vi "Modifying the Color Table2可加入多个颜色.vi"(7 "停止":bool, 8 "更新刻度颜色":bool, 9 "Z标尺.刻度值[]":cluster{"数值输入控件":dbl, "颜色盒":u32}[](array[cluster])=[{"数值输入控件"=0.0, "颜色盒"=16860}, {"数值输入控件"=7.0, "颜色盒"=2818033}, {"数值输入控件"=14.0, "颜色盒"=1244955}, {"数值输入控件"=21.0, "颜色盒"=16750634}, {"数值输入控件"=28.0, "颜色盒"=16711680}], 10 "高彩":u32(colorbox)=16711680, 11 "低彩":u32(colorbox)=11929) -> (3 "强度图":dbl[][](graph))   [LabVIEW 2015]
doc: "演示如何修改强度图或强度图表的色表。"
panel:
  out "强度图原":dbl[][](graph)
  in  "布尔":bool
  in  "插值率":dbl
  in  "显示范围":i32=64
  in  "数据范围":i32=64
  # "概述：演示如何修改强度图或强度图表的色表。\n操作步骤：\n1.运行VI。\n2.右键单击Z轴（图右边的颜色梯度）上的数字，选择刻度颜色，修改与刻度对应的颜色。观察颜色的变化，以及颜色变化对整个颜色梯度的影响。\n3.单击更新刻度颜色按钮，将新颜色应用于Z轴上的三个刻度。\n4.单击停止 停止VI运行。"
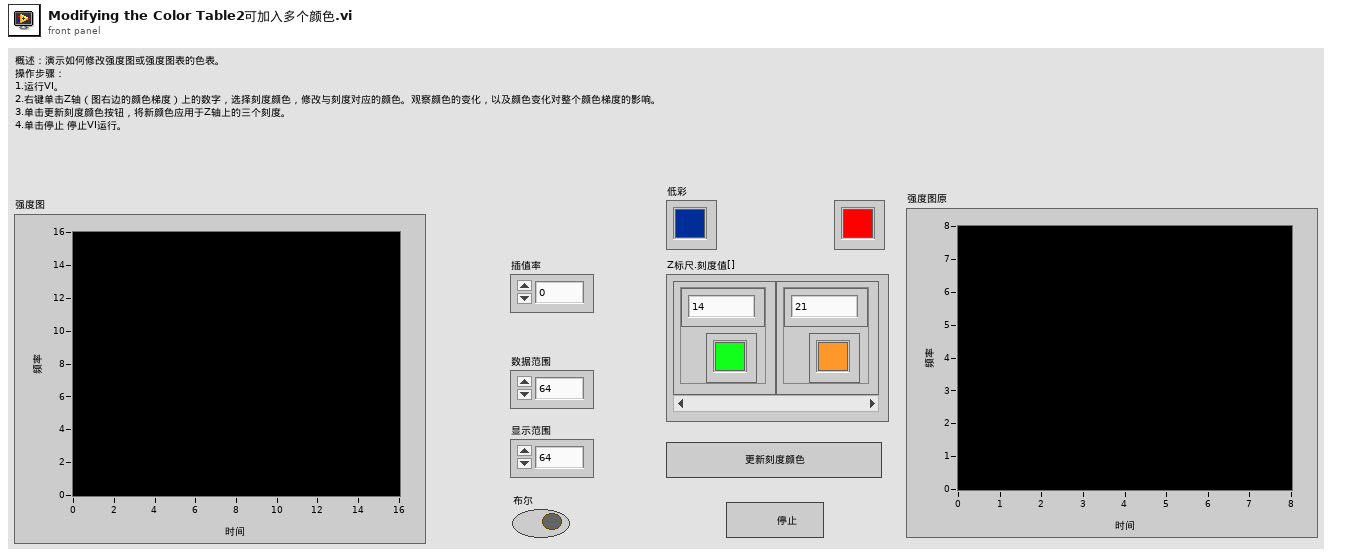
[diagram p1: front panel]
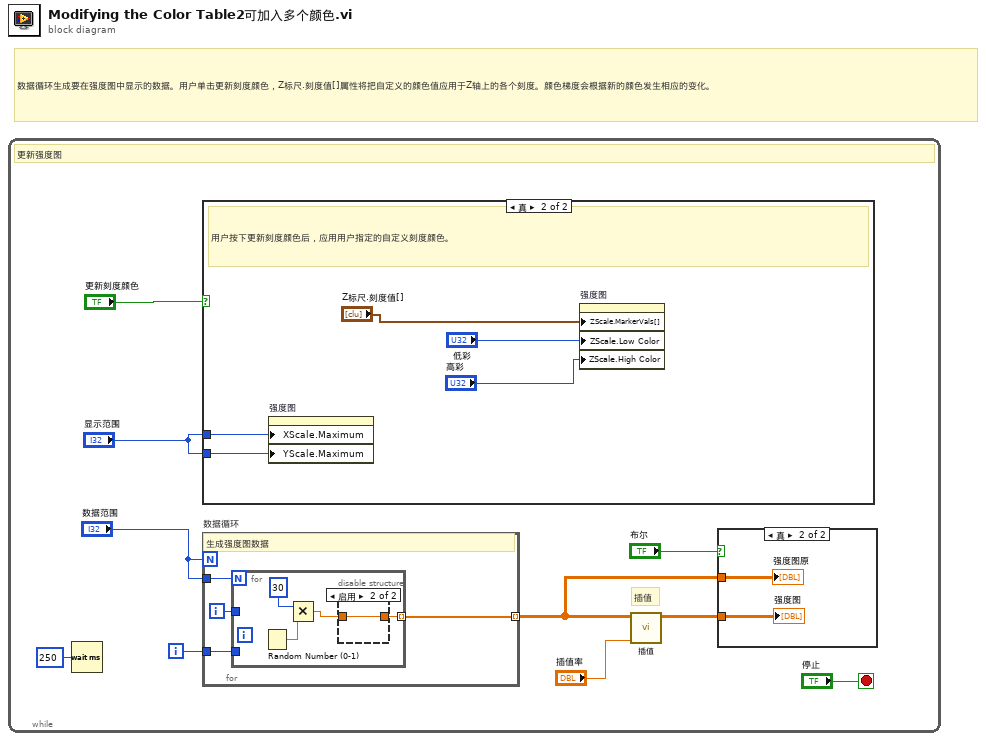
[diagram p0: block diagram]
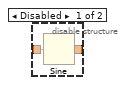
[diagram p4: hidden frame]
diagram:
  # "数据循环生成要在强度图中显示的数据。用户单击更新刻度颜色，Z标尺.刻度值[]属性将把自定义的颜色值应用于Z轴上的各个刻度。颜色梯度会根据新的颜色发生相应的变化。"
  n1 = while {
    i -> [w8]
    stop <- "停止" stop-if-true
    # "插值"
    # "更新强度图"
    n2 = Wait (ms)(milliseconds to wait=u32 250) -> ()  [unwired: 1 out]
    n3 = case shown="真" "更新刻度颜色" {
      tunnel: "显示范围" -> [_ w14]
      tunnel: "显示范围" -> [_ w13]
      frame False {
        # "如用户未按下更新刻度颜色，不对刻度颜色进行任何改变。"
      }
      frame True {
        # "用户按下更新刻度颜色后，应用用户指定的自定义刻度颜色。"
        n4 = property on="强度图" class="IntGraph (严格)"("XScale.Maximum"=w14, "YScale.Maximum"=w13) -> ()  [unwired: 2 in, 2 out]
        n5 = property on="强度图" class="强度图 (严格)"("ZScale.MarkerVals[]"="Z标尺.刻度值[]", "ZScale.Low Color"="低彩", "ZScale.High Color"="高彩") -> ()  [unwired: 2 in, 2 out]
      }
    }
    n6 = for "数据循环" {
      N: "数据范围" -> [_]
      tunnel: [w21] -> w1 mode=indexing
      tunnel: "数据范围" -> [w20]
      tunnel: w8 -> [w18]
      i -> [w19]
      # "生成强度图数据"
      n7 = for {
        N: w20 -> [_]
        tunnel: [w25] -> w21 mode=indexing
        tunnel: w19 -> [_]
        tunnel: w18 -> [_]
        n8 = Random Number (0-1)() -> (number: 0 to 1=w22:dbl)
        n9 = Multiply(x=30, y=w22) -> (x*y=w23:dbl)
        n10 = disable-structure shown="启用" {
          disable-tunnel: [w27 w28] -> w25
          disable-tunnel: w23 -> [w26 w28]
          frame Disabled {
            n11 = Sine(x=w26) -> (sin(x)=w27:dbl)
          }
          frame Enabled {
          }
        }
      }
    }
    n12 = call "插值.vi"("插值率"="插值率", "数字或点的数组"=w1) -> ("数字或点的数组输出"=w4:dbl[][])  [unwired: 8 in, 1 out]
    n13 = case shown="真" "布尔" {
      tunnel: w4 -> [_ w12]
      tunnel: w1 -> [_ w11]
      frame False {
      }
      frame True {
        "强度图" <- w12
        "强度图原" <- w11
      }
    }
  }
